vi "Get Root Actors.vi"(8 "error in (no error)":errorcluster, 11 "Monitor Data in":refnum<class "Monitor Data.lvclass">) -> (0 "error out":errorcluster, 2 "Root Actors":refnum<class "Message Enqueuer.lvclass">[](array[class]))   [LabVIEW 2017, in "MGI-Monitored Actor Core.lvlib" / "Monitor Data.lvclass"]
doc: "Returns the root level actors\n\nCopyright: MGI 2016\nAuthor: Derek Trepanier"
uses:
  Monitor Data.lvclass
  <vilib>/ActorFramework/Message Enqueuer/Message Enqueuer.lvclass
  Monitor Data.lvclass/Monitor Data.ctl
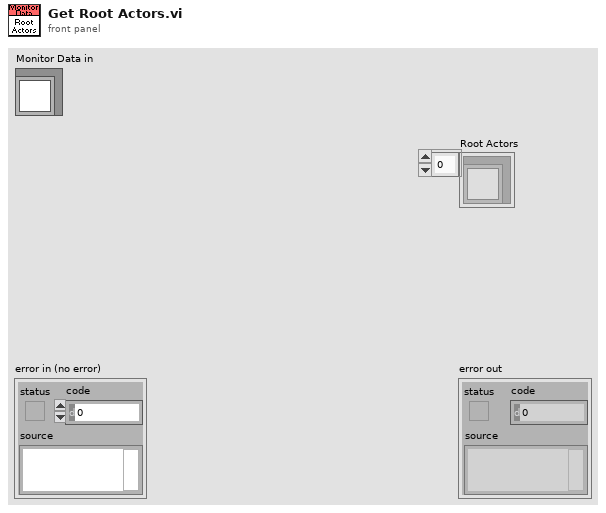
[diagram p1: front panel]
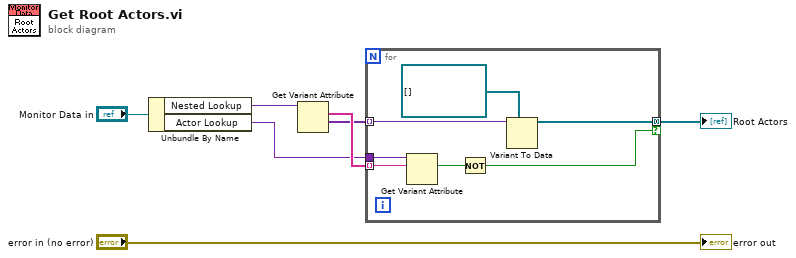
[diagram p0: block diagram]
diagram:
  n1 = Unbundle By Name("Monitor Data in") -> ("Nested Lookup"=w2:variant, "Actor Lookup"=w1:variant)
  n2 = Get Variant Attribute(Variant=w2) -> (names=w4:string[], values=w3:variant[])  [unwired: 3 in, 2 out]
  n3 = for {
    tunnel: w4 -> [w13] mode=indexing
    tunnel: [w9] -> w5 mode=concatenating if=w8
    tunnel: w3 -> [w11] mode=indexing
    tunnel: w1 -> [w14]
    n4 = Get Variant Attribute(Variant=w14, name=w13) -> (found=w12:bool)  [unwired: 2 in, 3 out]
    n5 = Not(x=w12) -> (.not. x?=w8:bool)
    n6 = Variant To Data(type=refnum<class "Message Enqueuer.lvclass">[] [], Variant=w11) -> (data=w9:refnum<class "Message Enqueuer.lvclass">[])  [unwired: 1 in, 1 out]
  }
  "Root Actors" <- w5
  "error out" <- "error in (no error)"
